vi "Initiate TS DAC.vi"(8 "error in":errorcluster, 11 "LNG Boiling Test Stand in":refnum<class "LNG Boiling Test Stand.lvclass">) -> (0 "error out":errorcluster, 3 "LNG Boiling Test Stand out":refnum<class "LNG Boiling Test Stand.lvclass">)   [LabVIEW 2019, in "Test Stands.lvlib" / "LNG Boiling Test Stand.lvclass"]
uses:
  LNG Boiling Test Stand.lvclass
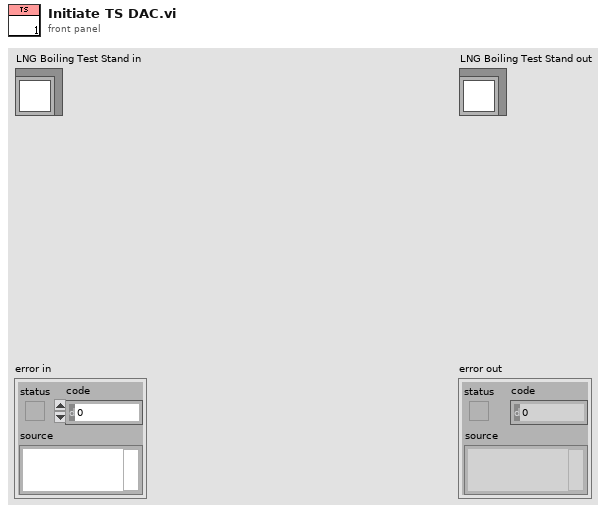
[diagram p1: front panel]
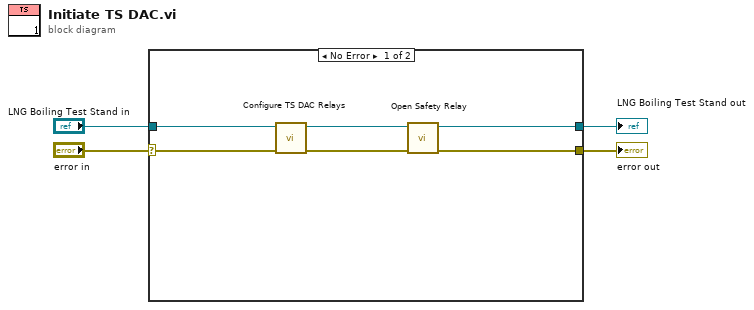
[diagram p0: block diagram]
diagram:
  n1 = case shown="No Error" "error in" {
    selector: "error in" -> [w7 w12]
    tunnel: [w5 w12] -> w4
    tunnel: [w8 w11] -> w3
    tunnel: "LNG Boiling Test Stand in" -> [w10 w11]
    frame No Error {
      n2 = call "Configure TS DAC Relays.vi"("error in"=w7, "LNG Boiling Test Stand in"=w10) -> ("error out"=w6:errorcluster, "LNG Boiling Test Stand out"=w9:refnum<class "LNG Boiling Test Stand.lvclass">)  [unwired: 8 in]
      n3 = call "Open Safety Relay.vi"("error in (no error)"=w6, "LNG Boiling Test Stand in"=w9) -> ("error out"=w5:errorcluster, "LNG Boiling Test Stand out"=w8:refnum<class "LNG Boiling Test Stand.lvclass">)  [unwired: 8 in]
    }
    frame Error {
    }
  }
  "error out" <- w4
  "LNG Boiling Test Stand out" <- w3
